vi "RW FF Array.vi"(0 "Refnum In":T2, 2 "Read (F)":bool, 7 "FFinfo In":T1(array[cluster]), 11 "Error In":errorcluster) -> (4 "Refnum Out":T2, 8 "FFinfo Out":T1(array[cluster]), 15 "Error Out":errorcluster)   [LabVIEW 2013]
uses:
  <vilib>/Utility/config.llb/Config Data RefNum.ctl
  <vilib>/Utility/config.llb/Write Key (Double).vi
  <vilib>/Utility/config.llb/Read Key (Double).vi
  <vilib>/Utility/config.llb/NI_LVConfig.lvlib
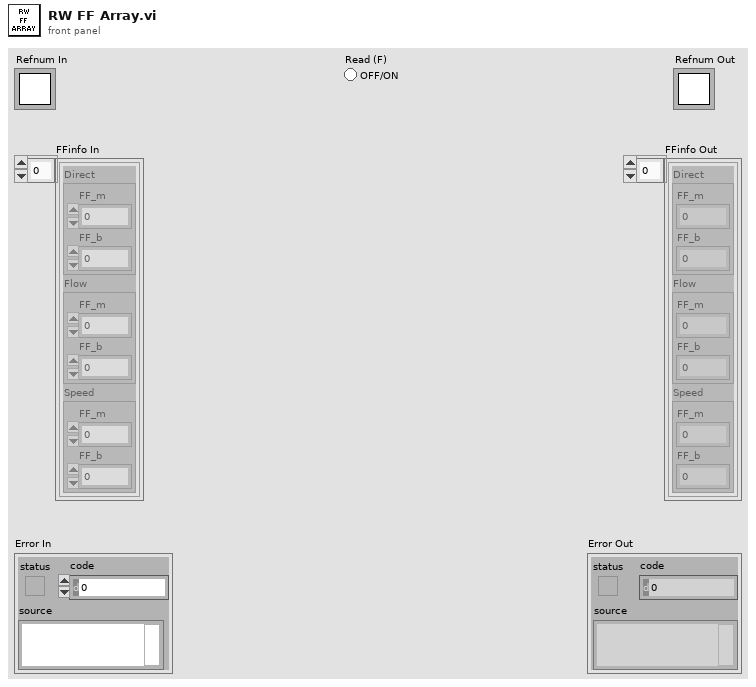
[diagram p1: front panel]
types:
  T1 = cluster{"Direct":cluster{"FF_m":dbl, "FF_b":dbl}, "Flow":cluster{"FF_m":dbl, "FF_b":dbl}, "Speed":cluster{"FF_m":dbl, "FF_b":dbl}}[]
  T2 = typedef "NI_LVConfig.lvlib/Config Data RefNum.ctl" = refnum<k1>
  T3 = cluster{"Direct":cluster{"FF_m":dbl, "FF_b":dbl}, "Flow":cluster{"FF_m":dbl, "FF_b":dbl}, "Speed":cluster{"FF_m":dbl, "FF_b":dbl}}
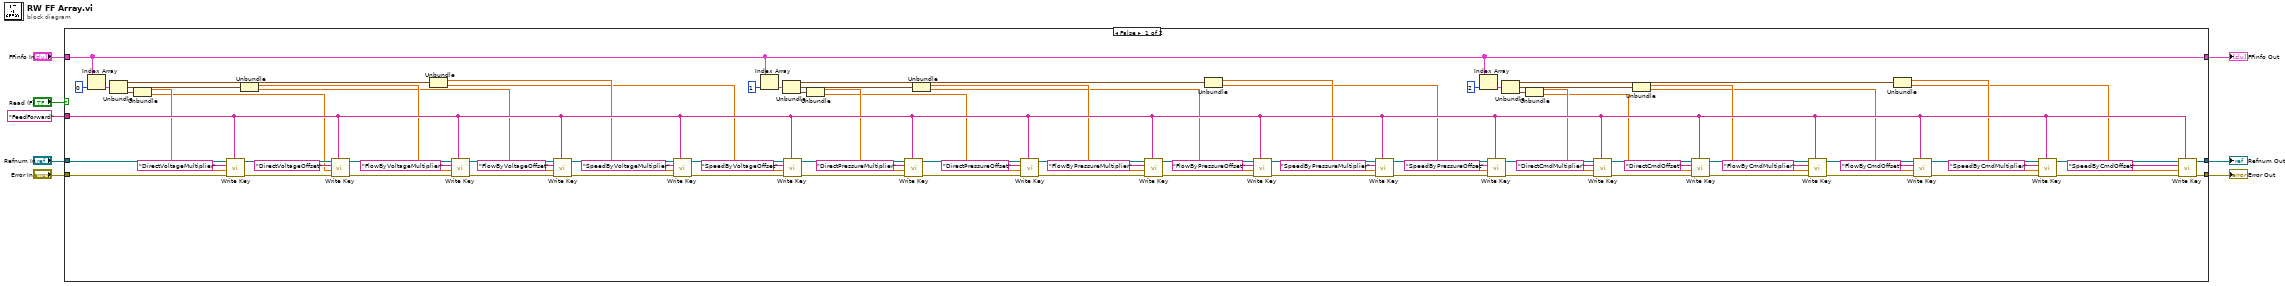
[diagram p0: block diagram]
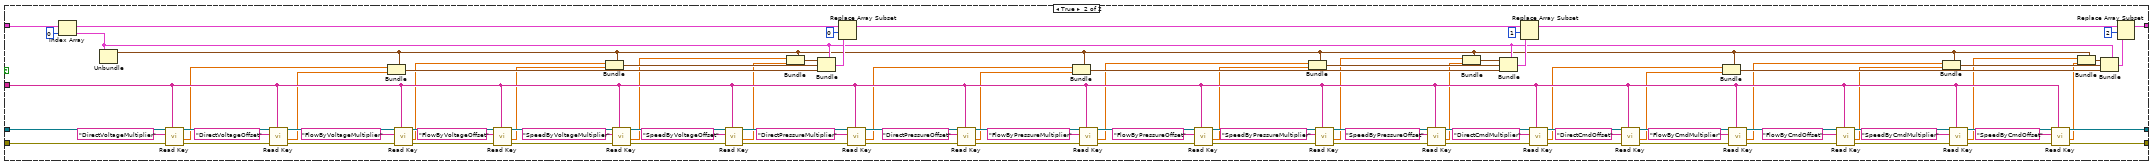
[diagram p2: hidden frame]
diagram:
  n1 = case shown="False" "Read (F)" {
    tunnel: "Error In" -> [w99 w195]
    tunnel: [w63 w153] -> w7
    tunnel: "Refnum In" -> [w90 w196]
    tunnel: [w62 w154] -> w4
    tunnel: "FeedForward" ("section") -> [w61 w152]
    tunnel: "FFinfo In" -> [w27 w135]
    tunnel: [w27 w118] -> w1
    frame False {
      n2 = Index Array(array=w27, index=0) -> (element=w41:T3)
      n3 = Unbundle(w41) -> ("Direct"=w40:cluster{"FF_m":dbl, "FF_b":dbl}, "Flow"=w38:cluster{"FF_m":dbl, "FF_b":dbl}, "Speed"=w39:cluster{"FF_m":dbl, "FF_b":dbl})
      n4 = Unbundle(w39) -> ("FF_m"=w26:dbl, "FF_b"=w25:dbl)
      n5 = call-poly <vilib>:"Write Key.vi"("section"=w61, "error in (no error)"=w99, "value"=w26, "key"="DirectVoltageMultiplier", "refnum"=w90) -> ("error out"=w98:errorcluster, "refnum out"=w89:T2)  [unwired: 4 in, 1 out]
      n6 = Unbundle(w38) -> ("FF_m"=w24:dbl, "FF_b"=w23:dbl)
      n7 = call-poly <vilib>:"Write Key.vi"("section"=w61, "error in (no error)"=w98, "value"=w25, "key"="DirectVoltageOffset", "refnum"=w89) -> ("error out"=w97:errorcluster, "refnum out"=w88:T2)  [unwired: 4 in, 1 out]
      n8 = Unbundle(w40) -> ("FF_m"=w22:dbl, "FF_b"=w21:dbl)
      n9 = call-poly <vilib>:"Write Key.vi"("section"=w61, "error in (no error)"=w97, "value"=w24, "key"="FlowByVoltageMultiplier", "refnum"=w88) -> ("error out"=w96:errorcluster, "refnum out"=w87:T2)  [unwired: 4 in, 1 out]
      n10 = call-poly <vilib>:"Write Key.vi"("section"=w61, "error in (no error)"=w96, "value"=w23, "key"="FlowByVoltageOffset", "refnum"=w87) -> ("error out"=w95:errorcluster, "refnum out"=w86:T2)  [unwired: 4 in, 1 out]
      n11 = call-poly <vilib>:"Write Key.vi"("section"=w61, "error in (no error)"=w95, "value"=w22, "key"="SpeedByVoltageMultiplier", "refnum"=w86) -> ("error out"=w94:errorcluster, "refnum out"=w85:T2)  [unwired: 4 in, 1 out]
      n12 = Index Array(array=w27, index=1) -> (element=w34:T3)
      n13 = Unbundle(w34) -> ("Direct"=w35:cluster{"FF_m":dbl, "FF_b":dbl}, "Flow"=w37:cluster{"FF_m":dbl, "FF_b":dbl}, "Speed"=w36:cluster{"FF_m":dbl, "FF_b":dbl})
      n14 = call-poly <vilib>:"Write Key.vi"("section"=w61, "error in (no error)"=w94, "value"=w21, "key"="SpeedByVoltageOffset", "refnum"=w85) -> ("error out"=w93:errorcluster, "refnum out"=w84:T2)  [unwired: 4 in, 1 out]
      n15 = Unbundle(w36) -> ("FF_m"=w20:dbl, "FF_b"=w19:dbl)
      n16 = call-poly <vilib>:"Write Key.vi"("section"=w61, "error in (no error)"=w93, "value"=w20, "key"="DirectPressureMultiplier", "refnum"=w84) -> ("error out"=w92:errorcluster, "refnum out"=w83:T2)  [unwired: 4 in, 1 out]
      n17 = Unbundle(w37) -> ("FF_m"=w18:dbl, "FF_b"=w17:dbl)
      n18 = call-poly <vilib>:"Write Key.vi"("section"=w61, "error in (no error)"=w92, "value"=w19, "key"="DirectPressureOffset", "refnum"=w83) -> ("error out"=w91:errorcluster, "refnum out"=w82:T2)  [unwired: 4 in, 1 out]
      n19 = call-poly <vilib>:"Write Key.vi"("section"=w61, "error in (no error)"=w91, "value"=w18, "key"="FlowByPressureMultiplier", "refnum"=w82) -> ("error out"=w65:errorcluster, "refnum out"=w64:T2)  [unwired: 4 in, 1 out]
      n20 = Unbundle(w35) -> ("FF_m"=w16:dbl, "FF_b"=w15:dbl)
      n21 = call-poly <vilib>:"Write Key.vi"("section"=w61, "error in (no error)"=w65, "value"=w17, "key"="FlowByPressureOffset", "refnum"=w64) -> ("error out"=w81:errorcluster, "refnum out"=w73:T2)  [unwired: 4 in, 1 out]
      n22 = call-poly <vilib>:"Write Key.vi"("section"=w61, "error in (no error)"=w81, "value"=w16, "key"="SpeedByPressureMultiplier", "refnum"=w73) -> ("error out"=w80:errorcluster, "refnum out"=w72:T2)  [unwired: 4 in, 1 out]
      n23 = Index Array(array=w27, index=2) -> (element=w31:T3)
      n24 = call-poly <vilib>:"Write Key.vi"("section"=w61, "error in (no error)"=w80, "value"=w15, "key"="SpeedByPressureOffset", "refnum"=w72) -> ("error out"=w79:errorcluster, "refnum out"=w71:T2)  [unwired: 4 in, 1 out]
      n25 = Unbundle(w31) -> ("Direct"=w30:cluster{"FF_m":dbl, "FF_b":dbl}, "Flow"=w28:cluster{"FF_m":dbl, "FF_b":dbl}, "Speed"=w29:cluster{"FF_m":dbl, "FF_b":dbl})
      n26 = Unbundle(w29) -> ("FF_m"=w14:dbl, "FF_b"=w13:dbl)
      n27 = call-poly <vilib>:"Write Key.vi"("section"=w61, "error in (no error)"=w79, "value"=w14, "key"="DirectCmdMultiplier", "refnum"=w71) -> ("error out"=w78:errorcluster, "refnum out"=w70:T2)  [unwired: 4 in, 1 out]
      n28 = Unbundle(w28) -> ("FF_m"=w12:dbl, "FF_b"=w11:dbl)
      n29 = call-poly <vilib>:"Write Key.vi"("section"=w61, "error in (no error)"=w78, "value"=w13, "key"="DirectCmdOffset", "refnum"=w70) -> ("error out"=w77:errorcluster, "refnum out"=w69:T2)  [unwired: 4 in, 1 out]
      n30 = call-poly <vilib>:"Write Key.vi"("section"=w61, "error in (no error)"=w77, "value"=w12, "key"="FlowByCmdMultiplier", "refnum"=w69) -> ("error out"=w76:errorcluster, "refnum out"=w68:T2)  [unwired: 4 in, 1 out]
      n31 = Unbundle(w30) -> ("FF_m"=w10:dbl, "FF_b"=w9:dbl)
      n32 = call-poly <vilib>:"Write Key.vi"("section"=w61, "error in (no error)"=w76, "value"=w11, "key"="FlowByCmdOffset", "refnum"=w68) -> ("error out"=w75:errorcluster, "refnum out"=w67:T2)  [unwired: 4 in, 1 out]
      n33 = call-poly <vilib>:"Write Key.vi"("section"=w61, "error in (no error)"=w75, "value"=w10, "key"="SpeedByCmdMultiplier", "refnum"=w67) -> ("error out"=w74:errorcluster, "refnum out"=w66:T2)  [unwired: 4 in, 1 out]
      n34 = call-poly <vilib>:"Write Key.vi"("section"=w61, "error in (no error)"=w74, "value"=w9, "key"="SpeedByCmdOffset", "refnum"=w66) -> ("error out"=w63:errorcluster, "refnum out"=w62:T2)  [unwired: 4 in, 1 out]
    }
    frame True {
      n35 = Index Array(array=w135, index=0) -> (element=w120:T3)
      n36 = Unbundle(w120) -> ("Direct"=w119:cluster{"FF_m":dbl, "FF_b":dbl})  [unwired: 2 out]
      n37 = call-poly <vilib>:"Read Key.vi"("section"=w152, "error in (no error)"=w195, "key"="DirectVoltageMultiplier", "refnum"=w196) -> ("error out"=w179:errorcluster, "value"=w100:dbl, "refnum out"=w194:T2)  [unwired: 4 in, 1 out]
      n38 = call-poly <vilib>:"Read Key.vi"("section"=w152, "error in (no error)"=w179, "key"="DirectVoltageOffset", "refnum"=w194) -> ("error out"=w180:errorcluster, "value"=w101:dbl, "refnum out"=w193:T2)  [unwired: 4 in, 1 out]
      n39 = Bundle(cluster=w119, "FF_m"=w100, "FF_b"=w101) -> (w136:cluster{"FF_m":dbl, "FF_b":dbl})
      n40 = call-poly <vilib>:"Read Key.vi"("section"=w152, "error in (no error)"=w180, "key"="FlowByVoltageMultiplier", "refnum"=w193) -> ("error out"=w181:errorcluster, "value"=w102:dbl, "refnum out"=w192:T2)  [unwired: 4 in, 1 out]
      n41 = call-poly <vilib>:"Read Key.vi"("section"=w152, "error in (no error)"=w181, "key"="FlowByVoltageOffset", "refnum"=w192) -> ("error out"=w182:errorcluster, "value"=w103:dbl, "refnum out"=w191:T2)  [unwired: 4 in, 1 out]
      n42 = Bundle(cluster=w119, "FF_m"=w102, "FF_b"=w103) -> (w137:cluster{"FF_m":dbl, "FF_b":dbl})
      n43 = call-poly <vilib>:"Read Key.vi"("section"=w152, "error in (no error)"=w182, "key"="SpeedByVoltageMultiplier", "refnum"=w191) -> ("error out"=w183:errorcluster, "value"=w104:dbl, "refnum out"=w190:T2)  [unwired: 4 in, 1 out]
      n44 = call-poly <vilib>:"Read Key.vi"("section"=w152, "error in (no error)"=w183, "key"="SpeedByVoltageOffset", "refnum"=w190) -> ("error out"=w184:errorcluster, "value"=w105:dbl, "refnum out"=w189:T2)  [unwired: 4 in, 1 out]
      n45 = Bundle(cluster=w119, "FF_m"=w104, "FF_b"=w105) -> (w138:cluster{"FF_m":dbl, "FF_b":dbl})
      n46 = Bundle(cluster=w120, "Direct"=w138, "Flow"=w137, "Speed"=w136) -> (w133:T3)
      n47 = Replace Array Subset(array=w135, new element=w133, index=0) -> (w121:T1)
      n48 = call-poly <vilib>:"Read Key.vi"("section"=w152, "error in (no error)"=w184, "key"="DirectPressureMultiplier", "refnum"=w189) -> ("error out"=w185:errorcluster, "value"=w106:dbl, "refnum out"=w188:T2)  [unwired: 4 in, 1 out]
      n49 = call-poly <vilib>:"Read Key.vi"("section"=w152, "error in (no error)"=w185, "key"="DirectPressureOffset", "refnum"=w188) -> ("error out"=w186:errorcluster, "value"=w107:dbl, "refnum out"=w187:T2)  [unwired: 4 in, 1 out]
      n50 = Bundle(cluster=w119, "FF_m"=w106, "FF_b"=w107) -> (w130:cluster{"FF_m":dbl, "FF_b":dbl})
      n51 = call-poly <vilib>:"Read Key.vi"("section"=w152, "error in (no error)"=w186, "key"="FlowByPressureMultiplier", "refnum"=w187) -> ("error out"=w156:errorcluster, "value"=w108:dbl, "refnum out"=w155:T2)  [unwired: 4 in, 1 out]
      n52 = call-poly <vilib>:"Read Key.vi"("section"=w152, "error in (no error)"=w156, "key"="FlowByPressureOffset", "refnum"=w155) -> ("error out"=w157:errorcluster, "value"=w109:dbl, "refnum out"=w172:T2)  [unwired: 4 in, 1 out]
      n53 = Bundle(cluster=w119, "FF_m"=w108, "FF_b"=w109) -> (w129:cluster{"FF_m":dbl, "FF_b":dbl})
      n54 = call-poly <vilib>:"Read Key.vi"("section"=w152, "error in (no error)"=w157, "key"="SpeedByPressureMultiplier", "refnum"=w172) -> ("error out"=w158:errorcluster, "value"=w110:dbl, "refnum out"=w171:T2)  [unwired: 4 in, 1 out]
      n55 = call-poly <vilib>:"Read Key.vi"("section"=w152, "error in (no error)"=w158, "key"="SpeedByPressureOffset", "refnum"=w171) -> ("error out"=w159:errorcluster, "value"=w111:dbl, "refnum out"=w170:T2)  [unwired: 4 in, 1 out]
      n56 = Bundle(cluster=w119, "FF_m"=w110, "FF_b"=w111) -> (w128:cluster{"FF_m":dbl, "FF_b":dbl})
      n57 = Bundle(cluster=w120, "Direct"=w128, "Flow"=w129, "Speed"=w130) -> (w132:T3)
      n58 = Replace Array Subset(array=w121, new element=w132, index=1) -> (w122:T1)
      n59 = call-poly <vilib>:"Read Key.vi"("section"=w152, "error in (no error)"=w159, "key"="DirectCmdMultiplier", "refnum"=w170) -> ("error out"=w160:errorcluster, "value"=w112:dbl, "refnum out"=w169:T2)  [unwired: 4 in, 1 out]
      n60 = call-poly <vilib>:"Read Key.vi"("section"=w152, "error in (no error)"=w160, "key"="DirectCmdOffset", "refnum"=w169) -> ("error out"=w161:errorcluster, "value"=w113:dbl, "refnum out"=w168:T2)  [unwired: 4 in, 1 out]
      n61 = Bundle(cluster=w119, "FF_m"=w112, "FF_b"=w113) -> (w125:cluster{"FF_m":dbl, "FF_b":dbl})
      n62 = call-poly <vilib>:"Read Key.vi"("section"=w152, "error in (no error)"=w161, "key"="FlowByCmdMultiplier", "refnum"=w168) -> ("error out"=w162:errorcluster, "value"=w115:dbl, "refnum out"=w167:T2)  [unwired: 4 in, 1 out]
      n63 = call-poly <vilib>:"Read Key.vi"("section"=w152, "error in (no error)"=w162, "key"="FlowByCmdOffset", "refnum"=w167) -> ("error out"=w163:errorcluster, "value"=w114:dbl, "refnum out"=w166:T2)  [unwired: 4 in, 1 out]
      n64 = Bundle(cluster=w119, "FF_m"=w115, "FF_b"=w114) -> (w126:cluster{"FF_m":dbl, "FF_b":dbl})
      n65 = call-poly <vilib>:"Read Key.vi"("section"=w152, "error in (no error)"=w163, "key"="SpeedByCmdMultiplier", "refnum"=w166) -> ("error out"=w164:errorcluster, "value"=w116:dbl, "refnum out"=w165:T2)  [unwired: 4 in, 1 out]
      n66 = call-poly <vilib>:"Read Key.vi"("section"=w152, "error in (no error)"=w164, "key"="SpeedByCmdOffset", "refnum"=w165) -> ("error out"=w153:errorcluster, "value"=w117:dbl, "refnum out"=w154:T2)  [unwired: 4 in, 1 out]
      n67 = Bundle(cluster=w119, "FF_m"=w116, "FF_b"=w117) -> (w127:cluster{"FF_m":dbl, "FF_b":dbl})
      n68 = Bundle(cluster=w120, "Direct"=w127, "Flow"=w126, "Speed"=w125) -> (w123:T3)
      n69 = Replace Array Subset(array=w122, new element=w123, index=2) -> (w118:T1)
    }
  }
  "Refnum Out" <- w4
  "Error Out" <- w7
  "FFinfo Out" <- w1
